vi "Free.vi"(8 "No Error":errorcluster, 11 "Mem [void *]":i64 format="%.0x") -> (0 "Error Out":errorcluster)   [LabVIEW 2026, in "SDL3.lvlib" / "Stdinc.lvlib"]
doc: "<B>LabVIEW Implementation</B>\nThis function works event in case of error in.\n\n<B>Summary</B>\nFree allocated memory.\n\n<B>Remarks</B>\nThe pointer is no longer valid after this call and cannot be dereferenced anymore.\n\nIf mem is NULL, this function does nothing."
uses:
  Stdinc.lvlib
  Lib/SDL3.dll
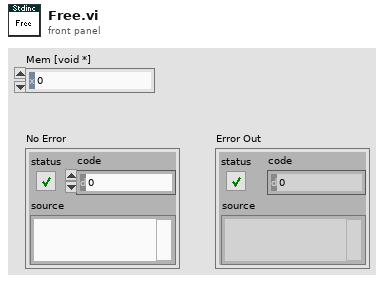
[diagram p1: front panel]
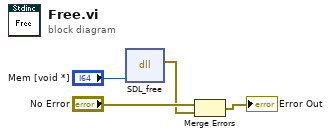
[diagram p0: block diagram]
diagram:
  n1 = dll-call lib="C:/Users/saukko/Dev/LV-SDL3/Sources/SDL3/Lib/SDL3.*" fn="SDL_free"("mem"="Mem [void *]") -> (error out=w1:errorcluster)  [unwired: 5 in, 1 out]
  n2 = Merge Errors("No Error", w1) -> (→"Error Out":errorcluster)
